vi "Write JSON Config.vi"(6 "Pretty Print?":bool, 8 "error in (no error)":errorcluster, 11 "AbsFunc_Two Term_DBL in":refnum<class "AbsFunc_Two Term_DBL.lvclass">) -> (0 "error out":errorcluster, 2 "JSON":string, 3 "AbsFunc_Two Term_DBL out":refnum<class "AbsFunc_Two Term_DBL.lvclass">)   [LabVIEW 2021, in "AbsFunc_Two Term_DBL.lvclass"]
uses:
  AbsFunc_Two Term_DBL.lvclass
  C:/Users/Tim/Documents/GitHub/LV_Abstract/Source/Abs_Types/Type/Abs_Type.lvclass
  AbsFunc_Two Term_DBL.lvclass/AbsFunc_Two Term_DBL.ctl
  <vilib>/Utility/LVClass/Get LV Class Name.vi
  Abs_Types/Double Float/Abs_Double Float.lvclass
  Abs_Types/Numeric/Abs_Numeric.lvclass
  Abs_Types/Type/Abs_Type.lvclass
  C:/Users/Tim/Documents/GitHub/LV_Abstract/Source/Abs_Types/Double Float/Abs_Double Float.lvclass
  C:/Users/Tim/Documents/GitHub/LV_Abstract/Source/Abs_Types/Floating Point/Abs_Floating Point.lvclass
  C:/Users/Tim/Documents/GitHub/LV_Abstract/Source/Abs_Types/Numeric/Abs_Numeric.lvclass
  C:/Users/Tim/Documents/GitHub/LV_Abstract/Source/Abs_Types/Value/Abs_Value.lvclass
  C:/Users/Tim/Documents/GitHub/LV_Abstract/Source/Functions/Support/Two Terminal/DBL/AbsFunc_Two Term_DBL.lvclass
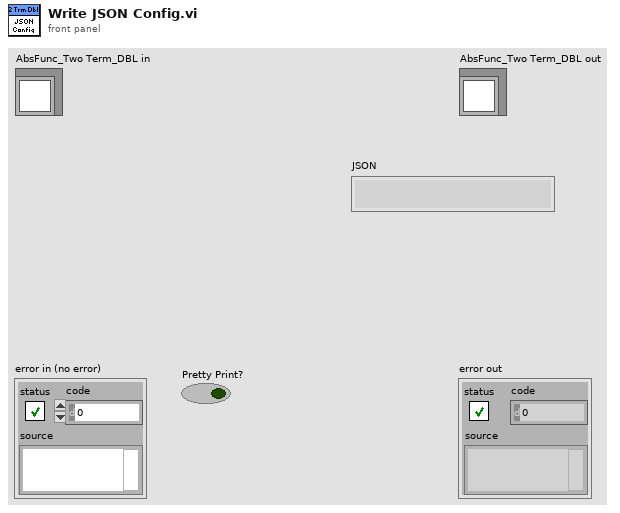
[diagram p1: front panel]
types:
  T1 = typedef "AbsFunc_Two Term_DBL.lvclass/Abstract Type.ctl" = refnum<class "Abs_Double Float.lvclass">
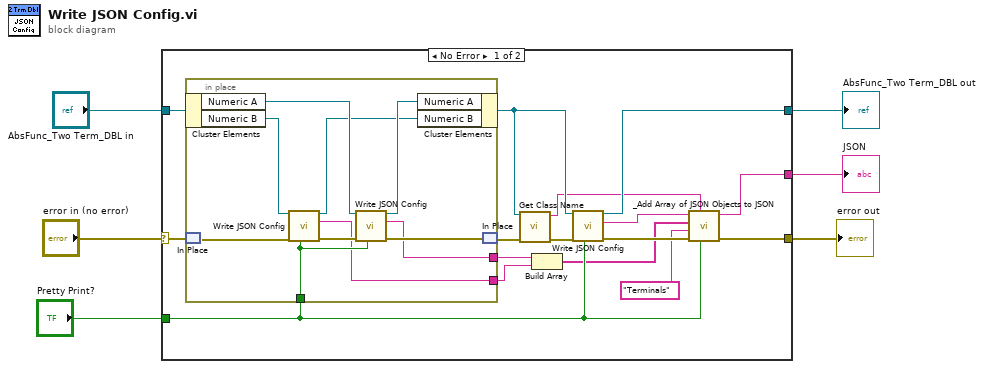
[diagram p0: block diagram]
diagram:
  n1 = case shown="No Error" "error in (no error)" {
    selector: "error in (no error)" -> [w17 w34]
    tunnel: "AbsFunc_Two Term_DBL in" -> [w22 w33]
    tunnel: [w21 w33] -> w5
    tunnel: [w13 _] -> w4
    tunnel: [w12 w34] -> w3
    tunnel: "Pretty Print?" -> [w11 _]
    frame No Error {
      n2 = in-place {
        in-place-border: w11 -> [w30]
        in-place-border: [w28] -> w20
        in-place-border: [w27] -> w19
        n3 = in-place-cluster #1(w22) -> ("Numeric A"=w26:T1, "Numeric B"=w24:refnum<class "Abs_Numeric.lvclass">)
        n4 = in-place-match #2(w17) -> (w31:errorcluster)
        n5 = call-dynamic "Write JSON Config.vi"("Pretty Print?"=w30, "error in (no error)"=w31, "Abs_Type in"=w24) -> ("error out"=w32:errorcluster, "JSON"=w27:string, "Abs_Type out"=w23:refnum<class "Abs_Numeric.lvclass">)  [unwired: 6 in]
        n6 = call-dynamic "Write JSON Config.vi"("Pretty Print?"=w30, "error in (no error)"=w32, "Abs_Type in"=w26) -> ("error out"=w29:errorcluster, "JSON"=w28:string, "Abs_Type out"=w25:T1)  [unwired: 6 in]
        n7 = in-place-cluster #1("Numeric A"=w25, "Numeric B"=w23) -> (w15:refnum<class "AbsFunc_Two Term_DBL.lvclass">)
        n8 = in-place-match #2(w29) -> (w18:errorcluster)
      }
      n9 = call "Get Class Name.vi"("error in (no error)"=w18, "Abs_Type in"=w15) -> ("error out"=w16:errorcluster, "class name"=w10:string)  [unwired: 8 in]
      n10 = Build Array(w20, w19) -> (w8:string[])
      n11 = call-parent "Write JSON Config.vi"("Pretty Print?"=w11, "error in (no error)"=w16, "Abs_Type in"=w15) -> ("error out"=w14:errorcluster, "JSON"=w9:string, "Abs_Type out"=w21:refnum<class "AbsFunc_Two Term_DBL.lvclass">)  [unwired: 6 in]
      n12 = call "_Add Array of JSON Objects to JSON.vi"("Pretty Print?"=w11, "JSON Object Name"=w10, "error in (no error)"=w14, "JSON Array Name"="Terminals", "JSON Objects"=w8, "JSON"=w9) -> ("error out"=w12:errorcluster, "<JSON>"=w13:string)  [unwired: 4 in]
    }
    frame Error {
    }
  }
  "error out" <- w3
  "AbsFunc_Two Term_DBL out" <- w5
  "JSON" <- w4
